vi "Untitled.vi"() -> ()   [LabVIEW 2020]
panel:
  in  "Tab Control":enum32{"Input"}(tab)
  in  "Pausa":bool
  out "Boolean":bool
  in  "Velocidad":dbl(knob) scale=1000.0..4000.0
  in  "Color leds":string(combo)
  in  "Visualización":enum32{"Ascendente", "Descendente"}(radio)
  in  "Base Numérica":string(combo)
  in  "Reset":bool
  out "Array":bool[][](array[boolean])
  out "Numero aleatorio k":dbl
  out "k en base 4":dbl
  out "k en base 11":dbl
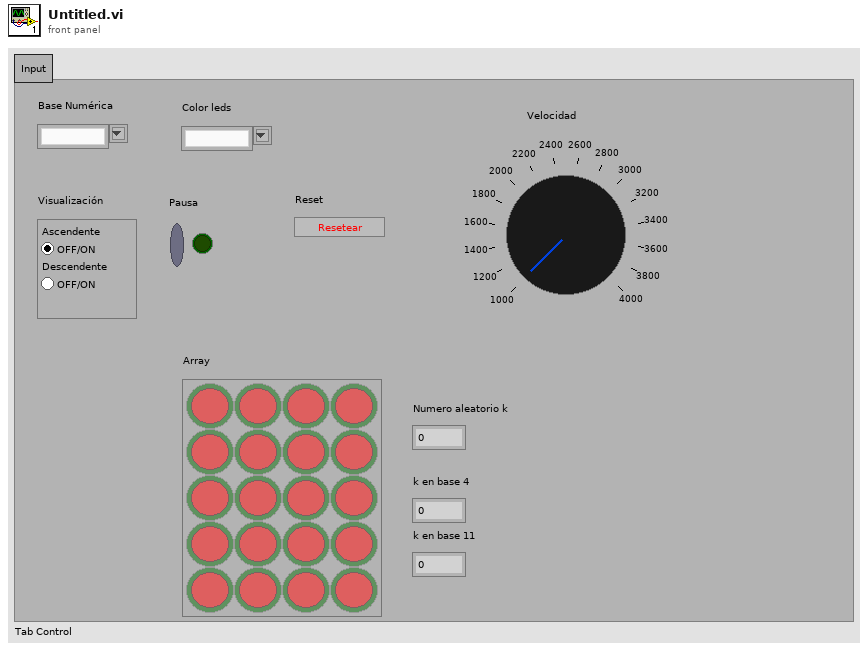
[diagram p1: front panel]
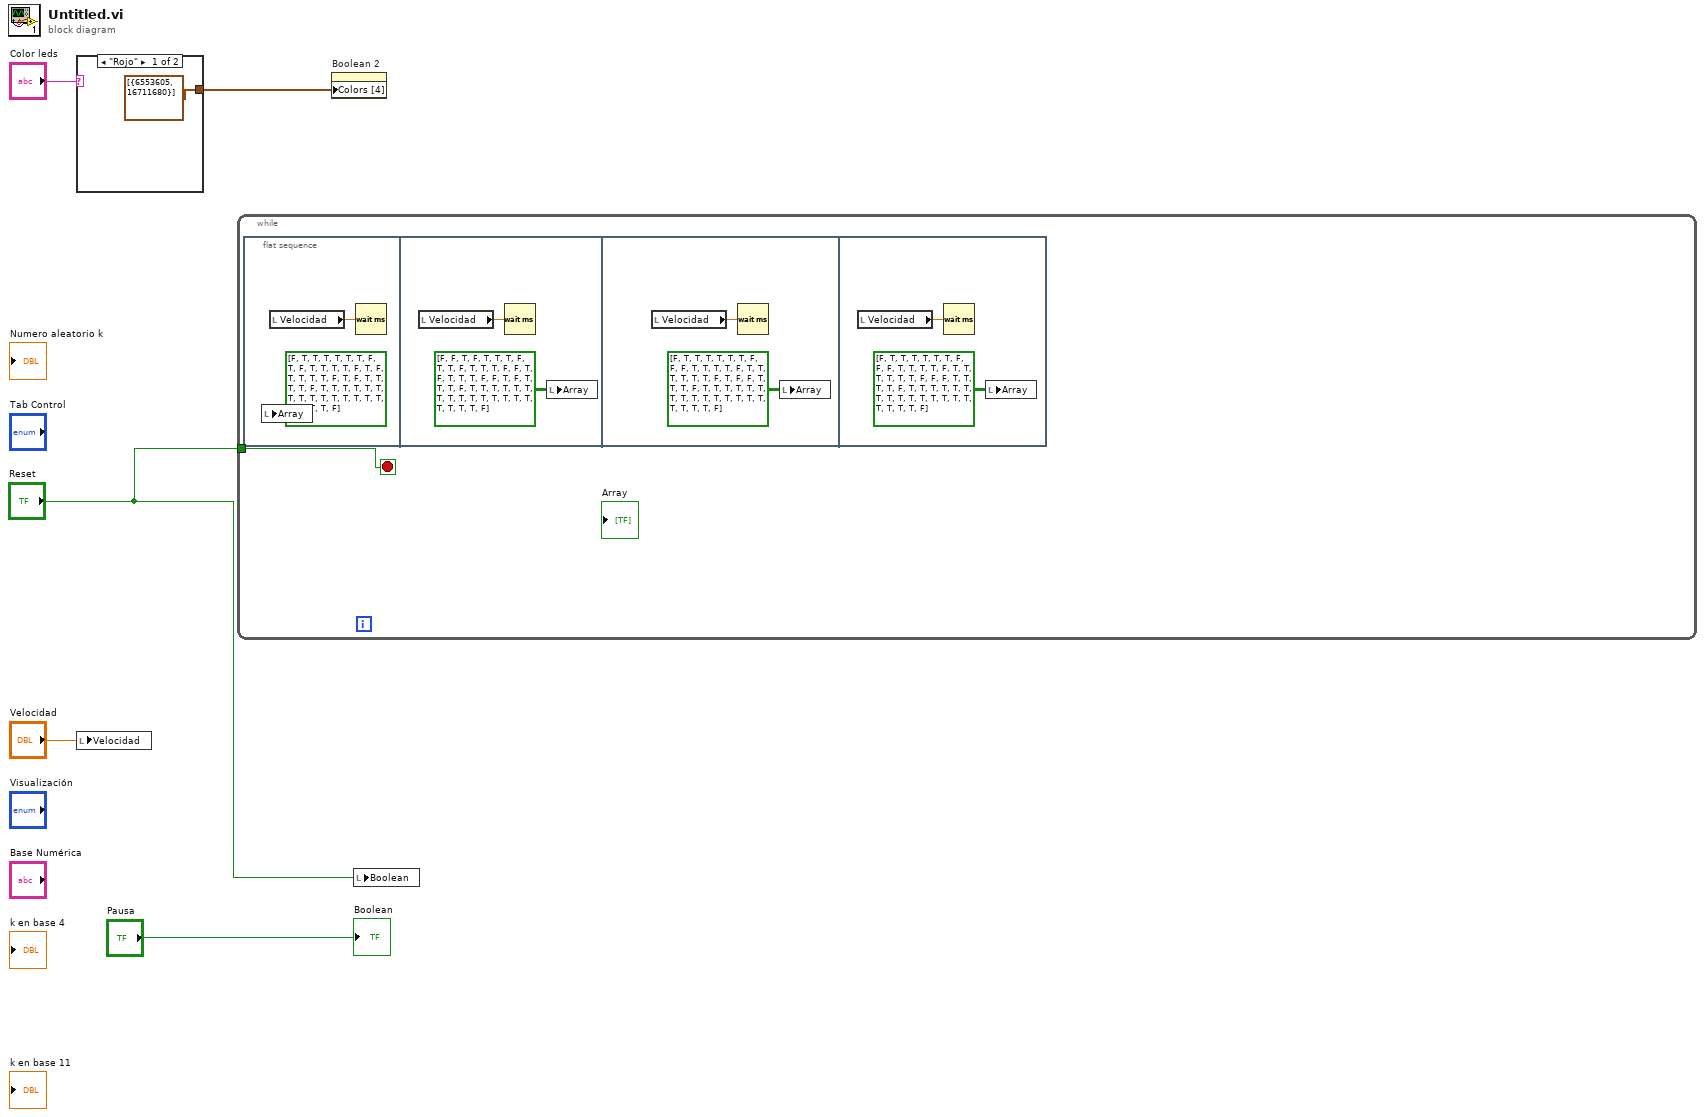
[diagram p0: block diagram]
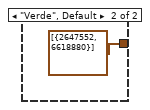
[diagram p2: hidden frame]
diagram:
  n1 = case shown="\"Rojo\"" "Color leds" {
    tunnel: [cluster{u32, u32}[] [{6553605, 16711680}] ("Colors [4]") cluster{u32, u32}[] [{2647552, 6618880}] ("Colors [4]")] -> w4
    frame "Rojo" {
    }
    frame "Verde", Default {
    }
  }
  n2 = local write "Velocidad"("Velocidad") -> ()
  n3 = while {
    tunnel: "Reset" -> [w8]
    stop <- w8 stop-if-true
    n4 = flat-sequence {
      frame #0 {
        n5 = local write "Array"(bool[][] [[FALSE, TRUE, TRUE, TRUE, TRUE, TRUE, TRUE], [FALSE, TRUE, FALSE, TRUE, TRUE, TRUE, TRUE], [FALSE, TRUE, FALSE, TRUE, TRUE, TRUE, TRUE], [FALSE, TRUE, FALSE, TRUE, TRUE, TRUE, TRUE], [FALSE, TRUE, TRUE, TRUE, TRUE, TRUE, TRUE], [TRUE, TRUE, TRUE, TRUE, TRUE, TRUE, TRUE], [TRUE, TRUE, TRUE, TRUE, TRUE, TRUE, FALSE]]) -> ()
        n6 = local read "Velocidad"() -> (w9:dbl)
        n7 = Wait (ms)(milliseconds to wait=w9) -> ()  [unwired: 1 out]
      }
      frame #1 {
        n8 = local read "Velocidad"() -> (w12:dbl)
        n9 = Wait (ms)(milliseconds to wait=w12) -> ()  [unwired: 1 out]
        n10 = local write "Array"(bool[][] [[FALSE, FALSE, TRUE, FALSE, TRUE, TRUE, TRUE], [FALSE, TRUE, TRUE, FALSE, TRUE, TRUE, TRUE], [FALSE, FALSE, TRUE, FALSE, TRUE, TRUE, TRUE], [FALSE, FALSE, TRUE, FALSE, TRUE, TRUE, TRUE], [FALSE, TRUE, TRUE, TRUE, TRUE, TRUE, TRUE], [TRUE, TRUE, TRUE, TRUE, TRUE, TRUE, TRUE], [TRUE, TRUE, TRUE, TRUE, TRUE, TRUE, FALSE]]) -> ()
      }
      frame #2 {
        n11 = local read "Velocidad"() -> (w13:dbl)
        n12 = Wait (ms)(milliseconds to wait=w13) -> ()  [unwired: 1 out]
        n13 = local write "Array"(bool[][] [[FALSE, TRUE, TRUE, TRUE, TRUE, TRUE, TRUE], [FALSE, FALSE, FALSE, TRUE, TRUE, TRUE, TRUE], [FALSE, TRUE, TRUE, TRUE, TRUE, TRUE, TRUE], [FALSE, TRUE, FALSE, FALSE, TRUE, TRUE, TRUE], [FALSE, TRUE, TRUE, TRUE, TRUE, TRUE, TRUE], [TRUE, TRUE, TRUE, TRUE, TRUE, TRUE, TRUE], [TRUE, TRUE, TRUE, TRUE, TRUE, TRUE, FALSE]]) -> ()
      }
      frame #3 {
        n14 = local read "Velocidad"() -> (w15:dbl)
        n15 = Wait (ms)(milliseconds to wait=w15) -> ()  [unwired: 1 out]
        n16 = local write "Array"(bool[][] [[FALSE, TRUE, TRUE, TRUE, TRUE, TRUE, TRUE], [FALSE, FALSE, FALSE, TRUE, TRUE, TRUE, TRUE], [FALSE, TRUE, TRUE, TRUE, TRUE, TRUE, TRUE], [FALSE, FALSE, FALSE, TRUE, TRUE, TRUE, TRUE], [FALSE, TRUE, TRUE, TRUE, TRUE, TRUE, TRUE], [TRUE, TRUE, TRUE, TRUE, TRUE, TRUE, TRUE], [TRUE, TRUE, TRUE, TRUE, TRUE, TRUE, FALSE]]) -> ()
      }
    }
  }
  n17 = property on="Boolean 2" class="Bool (strict)"("Colors [4]"=w4) -> ()  [unwired: 2 in, 2 out]
  n18 = local write "Boolean"("Reset") -> ()
  "Boolean" <- "Pausa"
